vi "Get Start Time.vi"(8 "error in (no error)":errorcluster, 11 "Log File in":refnum<class "Log File.lvclass">) -> (0 "error out":errorcluster, 2 "Start Time":timestamp, 3 "Log File out":refnum<class "Log File.lvclass">)   [LabVIEW 2012, in "Waveform Data Logger Engine.lvlib" / "Log File.lvclass"]
uses:
  Log File.lvclass
  Log File.lvclass/Log File.ctl
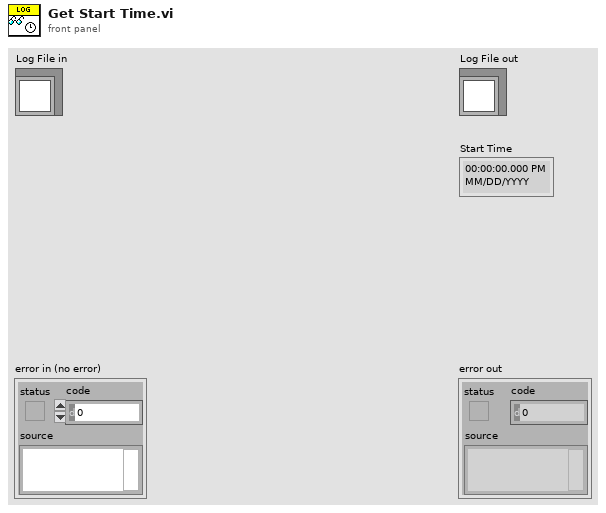
[diagram p1: front panel]
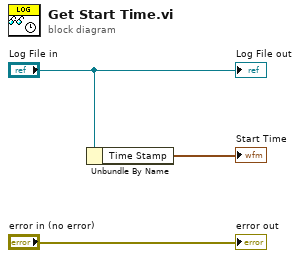
[diagram p0: block diagram]
diagram:
  n1 = Unbundle By Name("Log File in") -> ("Time Stamp"=→"Start Time":timestamp)
  "error out" <- "error in (no error)"
  "Log File out" <- "Log File in"
